vi "CreateMessageQueue.vi"(4 "initial message values":string[](array[string]), 5 "initial message names":string[](array[string]), 6 "error in":errorcluster, 8 "max size (-1)":i32=-1, 9 "message queue name":string) -> (0 "error out":errorcluster, 1 "timed out":bool[](array[boolean]), 3 "message queue out":T1)   [LabVIEW 2014, in "Raspberry Pi Compatible Compiler for LabVIEW.lvlib" / "SimpleMessaging.lvlib"]
uses:
  SimpleMessaging.lvlib
  MessageQueueTD.ctl
  MessageTD.ctl
panel:
  in  "timeout in ms (-1)":i32
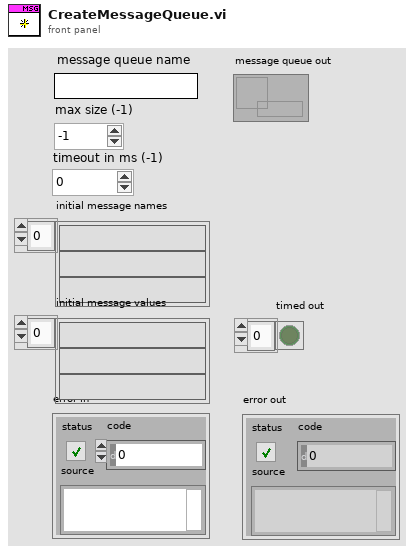
[diagram p1: front panel]
types:
  T1 = typedef "Raspberry Pi Compatible Compiler for LabVIEW.lvlib/SimpleMessaging.lvlib/MessageQueueTD.ctl" = refnum<queue>
  T2 = typedef "Raspberry Pi Compatible Compiler for LabVIEW.lvlib/SimpleMessaging.lvlib/MessageTD.ctl" = cluster{"Name":string, "Value":string}
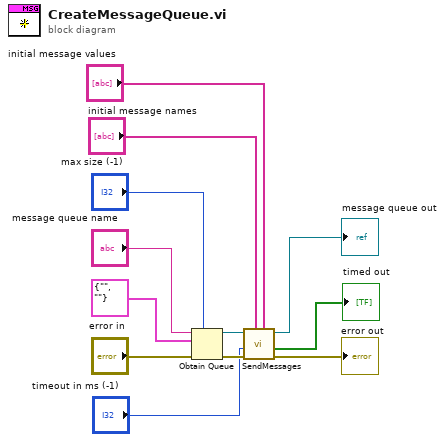
[diagram p0: block diagram]
diagram:
  n1 = Obtain Queue(max queue size (-1, unlimited)="max size (-1)", name (unnamed)="message queue name", element data type=T2 {"Name"="", "Value"=""} ("Message"), error in (no error)="error in") -> (queue out=w8:refnum<queue>, error out=w6:errorcluster)  [unwired: 1 in, 1 out]
  n2 = call "SendMessages.vi"("message values"="initial message values", "message names"="initial message names", "error in"=w6, "timeout in ms (-1)"="timeout in ms (-1)", "message queue in"=w8) -> ("error out"=→"error out":errorcluster, "timed out"=→"timed out":bool[], "message queue out"=→"message queue out":T1)  [unwired: 2 in]
